vi "PIV_scale.vi"(8 "error in (no error)":errorcluster, 9 "Scaling":cluster{"dt (sec)":dbl, "pixels/mm":dbl}, 10 "Add Velocity":cluster{"u":i32, "v":i32}, 11 "interpolated":T1) -> (0 "error out":errorcluster, 3 "velocities":T1)   [LabVIEW 2025]
uses:
  PIV_velocities.ctl
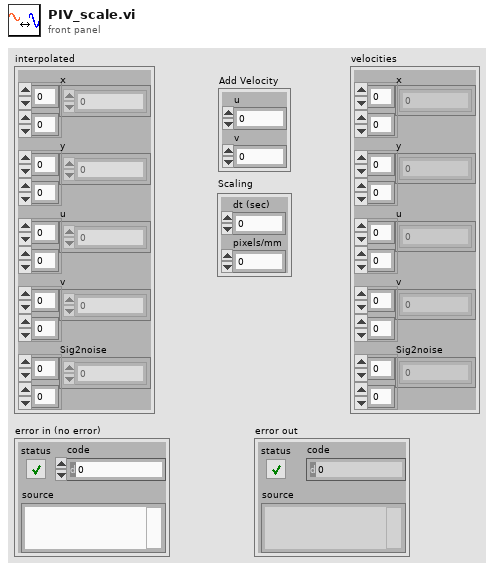
[diagram p1: front panel]
types:
  T1 = typedef "PIV_velocities.ctl" = cluster{"x":dbl[][], "y":dbl[][], "u":dbl[][], "v":dbl[][], "Sig2noise":dbl[][]}
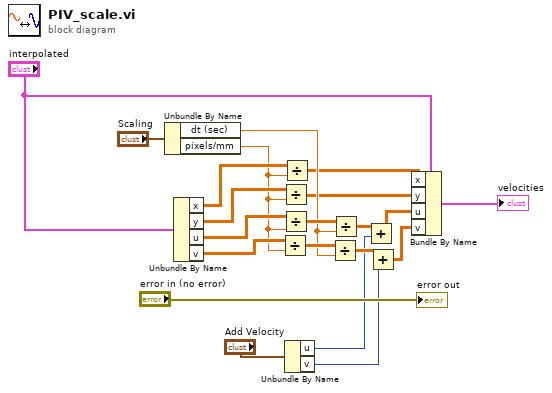
[diagram p0: block diagram]
diagram:
  n1 = Unbundle By Name("Scaling") -> ("dt (sec)"=w12:dbl, "pixels/mm"=w15:dbl)
  n2 = Unbundle By Name("interpolated") -> ("x"=w19:dbl[][], "y"=w18:dbl[][], "u"=w17:dbl[][], "v"=w16:dbl[][])
  n3 = Divide(x=w16, y=w15) -> (x/y=w13:dbl[][])
  n4 = Divide(x=w18, y=w15) -> (x/y=w9:dbl[][])
  n5 = Divide(x=w17, y=w15) -> (x/y=w14:dbl[][])
  n6 = Divide(x=w19, y=w15) -> (x/y=w10:dbl[][])
  n7 = Unbundle By Name("Add Velocity") -> ("u"=w3:i32, "v"=w1:i32)
  n8 = Divide(x=w13, y=w12) -> (x/y=w7:dbl[][])
  n9 = Divide(x=w14, y=w12) -> (x/y=w5:dbl[][])
  n10 = Add(x=w5, y=w3) -> (x+y=w4:dbl[][])
  n11 = Add(x=w7, y=w1) -> (x+y=w2:dbl[][])
  n12 = Bundle By Name(cluster="interpolated", "x"=w10, "y"=w9, "u"=w4, "v"=w2) -> (→"velocities":T1)
  "error out" <- "error in (no error)"
